vi "Lab4.vi"() -> ()   [LabVIEW 2012]
uses:
  <instrlib>/niUSRP/niUSRP Write Tx Data (CDB).vi
panel:
  in  "waveform size":i32
  in  "stop":bool
  out "error out":errorcluster
  out "coerced gain":dbl format="%#_6f"
  out "coerced carrier frequency":dbl=100000.0 format="%#_6p"
  out "coerced IQ rate":dbl=100000.0 format="%#_6p"
  in  "active antenna":string
  in  "gain":dbl format="%#_6f"
  in  "carrier frequency":dbl=100000.0 format="%#_6p"
  in  "IQ rate":dbl=100000.0 format="%#_6p"
  in  "USRP IP Address":refnum<k15>
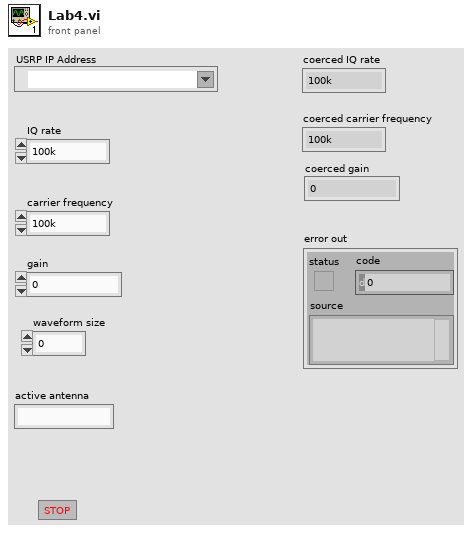
[diagram p1: front panel]
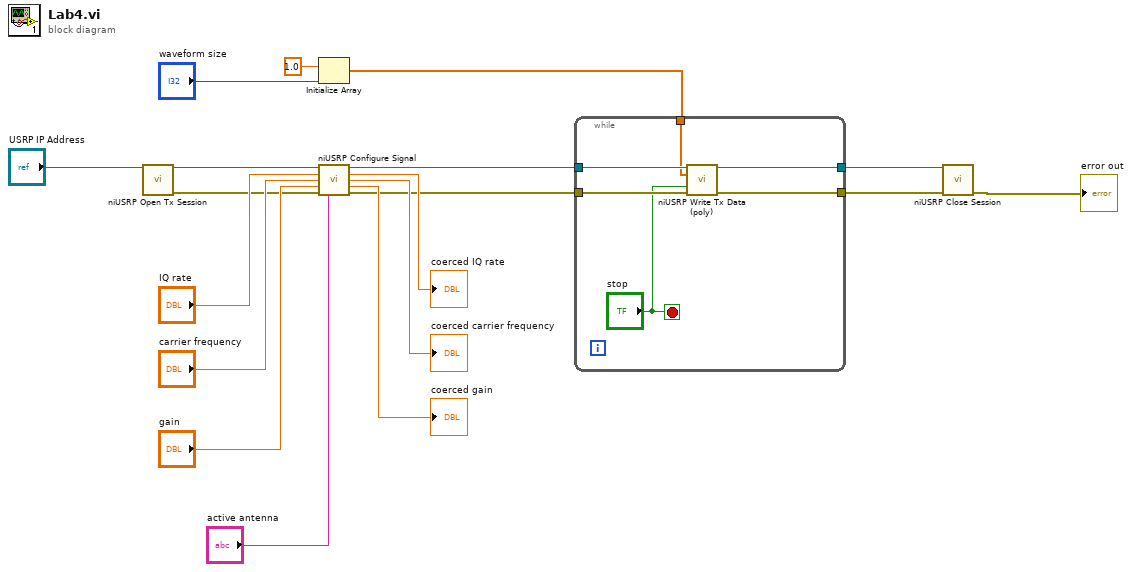
[diagram p0: block diagram]
diagram:
  n1 = call <instrlib>:"niUSRP Open Tx Session.vi"("device names"="USRP IP Address") -> ("session handle out"=w17:refnum<k15>, "error out"=w8:errorcluster)  [unwired: 13 in]
  n2 = Initialize Array(1.0 ("element"), "waveform size") -> (w2:dbl[])
  n3 = call <instrlib>:"niUSRP Configure Signal.vi"("session handle"=w17, "IQ rate"="IQ rate", "carrier frequency"="carrier frequency", "gain"="gain", "error in (no error)"=w8, "active antenna"="active antenna") -> ("session handle out"=w9:refnum<k15>, "coerced IQ rate"=→"coerced IQ rate":dbl, "coerced carrier frequency"=→"coerced carrier frequency":dbl, "coerced gain"=→"coerced gain":dbl, "error out"=w7:errorcluster)  [unwired: 5 in]
  n4 = while {
    tunnel: w9 -> [w24]
    tunnel: w7 -> [w23]
    tunnel: [w22] -> w6
    tunnel: [w20] -> w4
    tunnel: w2 -> [w19]
    stop <- "stop" stop-if-true
    n5 = call-poly <instrlib>:"niUSRP Write Tx Data (poly).vi"("session handle"=w24, "data"=w19, "end of data?"="stop", "error in (no error)"=w23) -> ("session handle out"=w20:refnum<k15>, "error out"=w22:errorcluster)  [unwired: 10 in]
  }
  n6 = call <instrlib>:"niUSRP Close Session.vi"("session handle"=w4, "error in (no error)"=w6) -> ("error out"=→"error out":errorcluster)  [unwired: 13 in]
